vi "Autonomous No Shift 1 Tote 1 Container.vi"(11 "Cluster":T2={"Move Speed"=0.0, "Turning Speed"=0.53, "Arm speed"=0.0, "Desired Arm height (lift)"=17.0, "Initial Turn (Degrees)"=-18.0, "Desired Arm height (lowered)"=-12.0, "Drive Forward Time"=0.0, "Turn Degrees"=-130.0, "Position Speed"=0.3, "2nd Lift Height"=10.0}) -> ()   [LabVIEW 2014]
uses:
  Backup Auto States.ctl
  Robot Global Data.vi
  Desired Arm Position.vi
  <vilib>/Rock Robotics/WPI/RobotDrive/WPI_RobotDriveGetSetRefNum.vi
  <vilib>/Rock Robotics/WPI/RobotDrive/WPI_RobotDriveArcadeDrive_Standard(NoSaturation).vi
panel:
  in  "End Position?":bool
  out "Enum":T1=enum."Stop"
  in  "Range":dbl=2.0
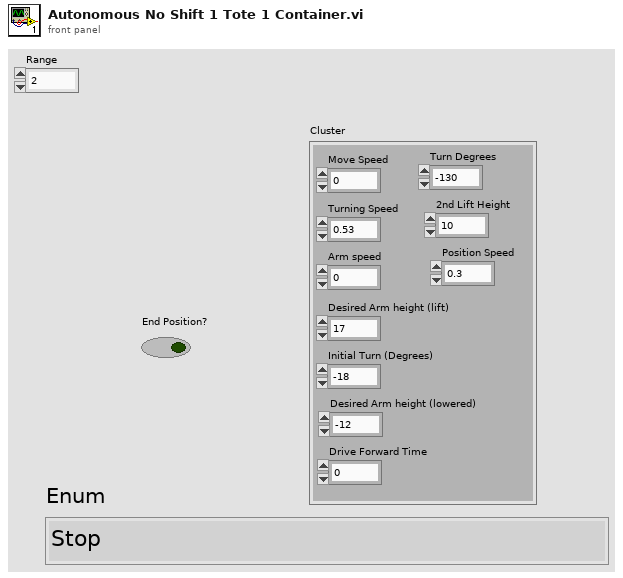
[diagram p1: front panel]
types:
  T1 = typedef "Backup Auto States.ctl" = enum16{"Start", "Grab container", "Lift arms", "Move to position", "Position robot", "Let go of container + Lower Arms", "Lift tote and container", "Turn towards S.P.", "Move forward", "Turn After hitting S.P.", "Move Until S.P. is gone", "Turn towards Auto Zone", "Drive to Auto Zone", "Stop"}
  T2 = cluster{"Move Speed":dbl, "Turning Speed":dbl, "Arm speed":dbl, "Desired Arm height (lift)":dbl, "Initial Turn (Degrees)":dbl, "Desired Arm height (lowered)":dbl, "Drive Forward Time":dbl, "Turn Degrees":dbl, "Position Speed":dbl, "2nd Lift Height":dbl}
  T3 = typedef "WPI_DigitalInputDevRef.ctl" = cluster{"DevStatus":errorcluster, "DIO Channel":T4, "Controller":T5}
  T4 = typedef "FPGA_DIOChannel.ctl" = enum8{"DIO 0", "DIO 1", "DIO 2", "DIO 3", "DIO 4", "DIO 5", "DIO 6", "DIO 7", "DIO 8", "DIO 9", "DIO MXP 0", "DIO MXP 1", "DIO MXP 2", "DIO MXP 3", "DIO MXP 4", "DIO MXP 5", "DIO MXP 6", "DIO MXP 7", "DIO MXP 8", "DIO MXP 9", "DIO MXP 10", "DIO MXP 11", "DIO MXP 12", "DIO MXP 13", "DIO MXP 14", "DIO MXP 15", "Invalid"}
  T5 = typedef "FPGA_TypedefDigitalModule.ctl" = enum16{"Controller 1"}
  T6 = typedef "WPI_RobotDriveDevRef.ctl" = cluster{"DevStatus":errorcluster, "Motors[]":T7[], "Square Inputs":bool, "Max Output":dbl}
  T7 = typedef "WPI_MotorControlDeviceRef.ctl" = cluster{"DeviceStatus":errorcluster, "Type":T8, "PWM":cluster{"Controller":T5, "PWM Channel":T9, "DeadBand":T10}, "CAN":cluster{"Device Number":u8, "Control Mode":T11, "Semaphore":T12, "Max Vout":dbl, "TalonSRX Control Mode":T13}, "Invert":bool, "TransformRef":T14, "InvTransformRef":T14}
  T8 = typedef "WPI_MotorControlType.ctl" = enum16{"PWM", "CAN", "CANTalonSRX"}
  T9 = typedef "FPGA_DIOPWMChannel.ctl" = enum8{"PWM 0", "PWM 1", "PWM 2", "PWM 3", "PWM 4", "PWM 5", "PWM 6", "PWM 7", "PWM 8", "PWM 9", "PWM MXP 0", "PWM MXP 1", "PWM MXP 2", "PWM MXP 3", "PWM MXP 4", "PWM MXP 5", "PWM MXP 6", "PWM MXP 7", "PWM MXP 8", "PWM MXP 9", "Invalid"}
  T10 = typedef "WPI_PWMDeadband.ctl" = cluster{"Name":string, "maxPositivePwm":i32, "minPositivePwm":i32, "centerPwm":i32, "maxNegativePwm":i32, "minNegativePwm":i32, "angularRange":u16}
  T11 = typedef "WPI_CANJaguar_ControlMode.ctl" = enum8{"Percent VBus", "Current", "Speed", "Position", "Voltage"}
  T12 = typedef "Semaphore RefNum" = refnum<k1>
  T13 = typedef "WPI_CANTalonSRX_APIControlMode.ctl" = enum8{"Percent VBus", "Speed", "Position", "Slave", "Unchanged / Invalid"}
  T14 = typedef "WPI_PWMTransform_ConPane.ctl" = refnum<vi>
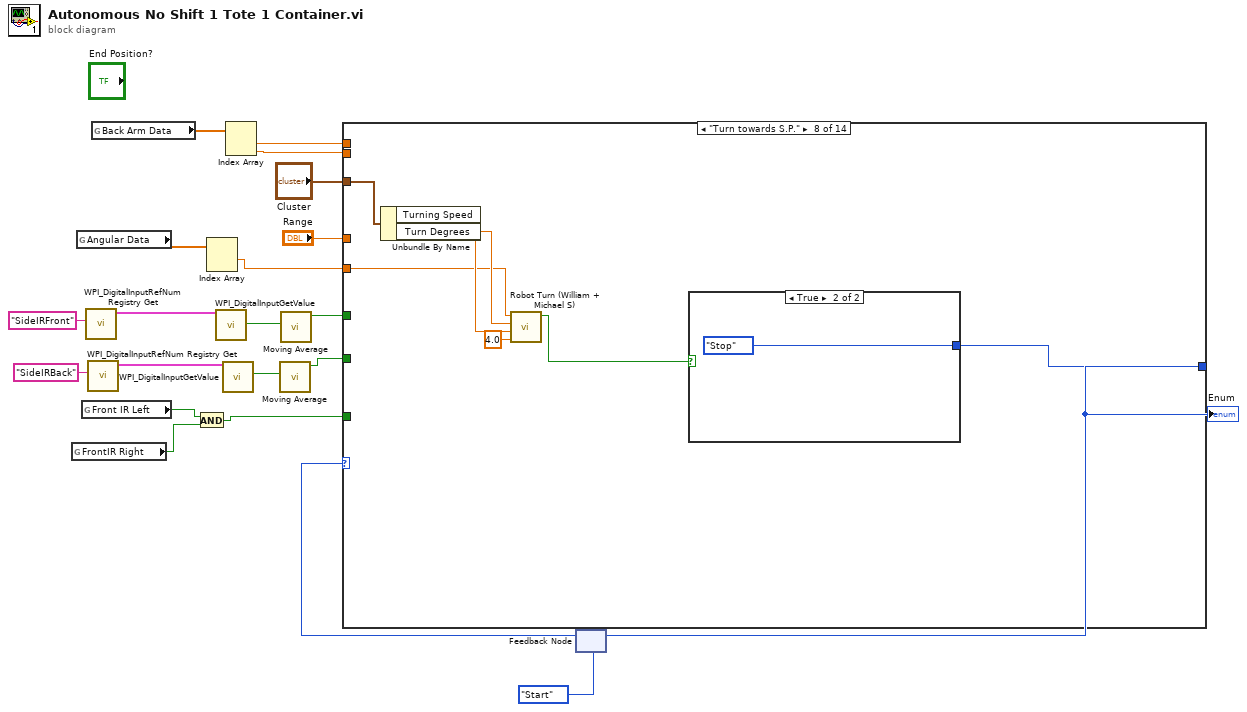
[diagram p0: block diagram]
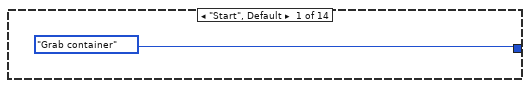
[diagram p2: hidden frame]
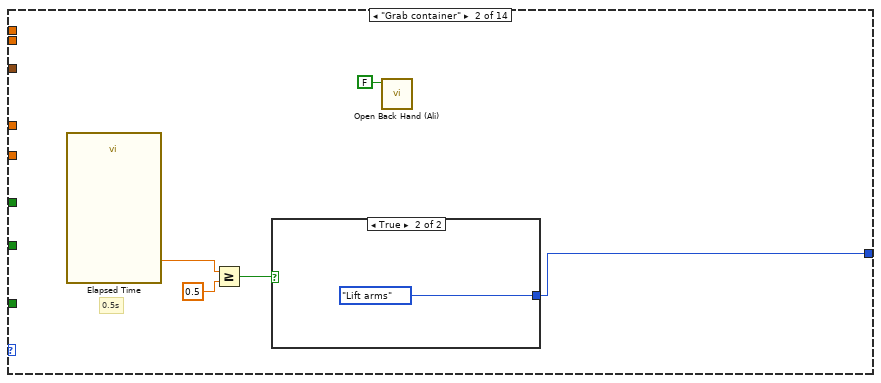
[diagram p3: hidden frame]
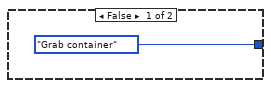
[diagram p4: hidden frame]
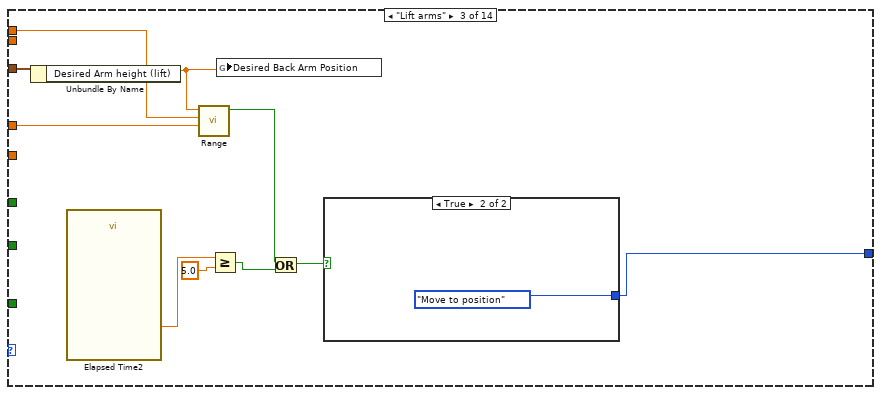
[diagram p5: hidden frame]
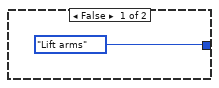
[diagram p6: hidden frame]
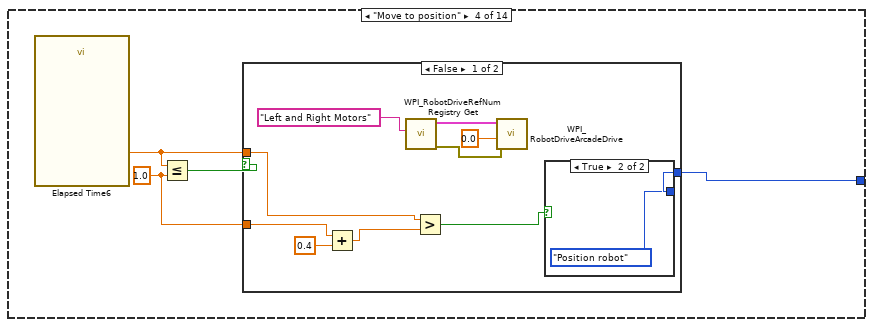
[diagram p7: hidden frame]
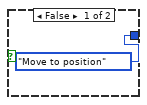
[diagram p8: hidden frame]
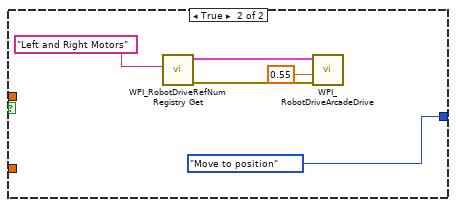
[diagram p9: hidden frame]
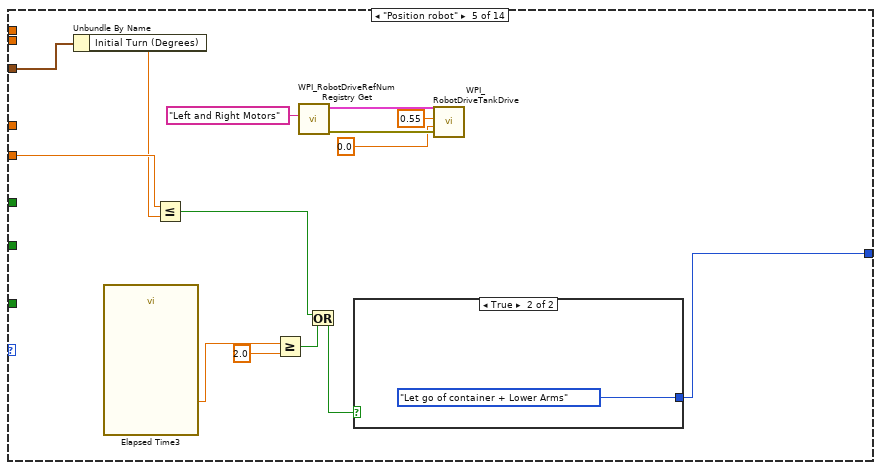
[diagram p10: hidden frame]
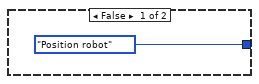
[diagram p11: hidden frame]
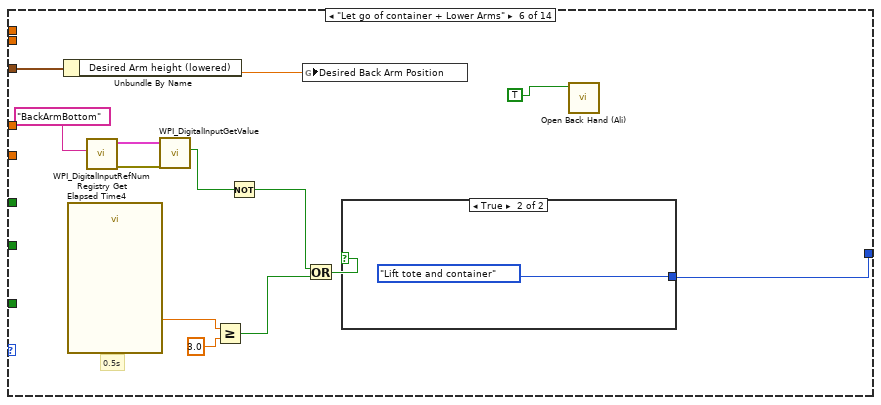
[diagram p12: hidden frame]
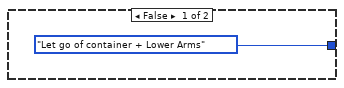
[diagram p13: hidden frame]
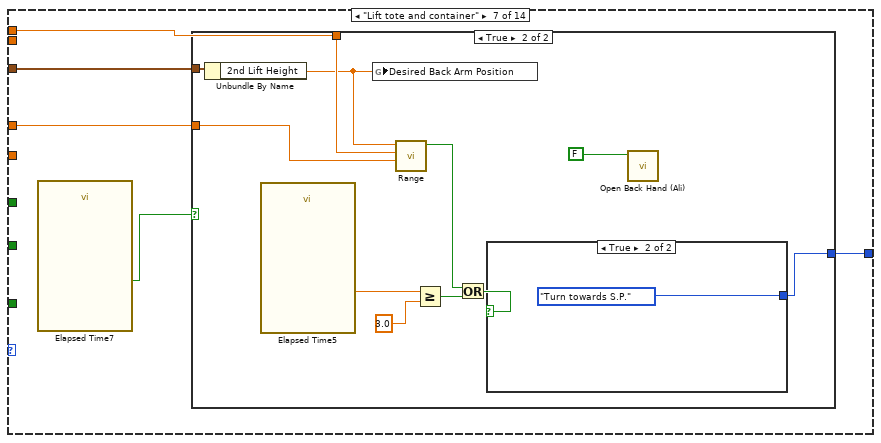
[diagram p14: hidden frame]
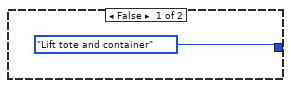
[diagram p15: hidden frame]
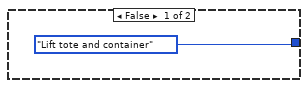
[diagram p16: hidden frame]
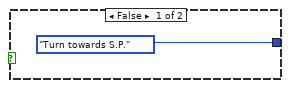
[diagram p17: hidden frame]
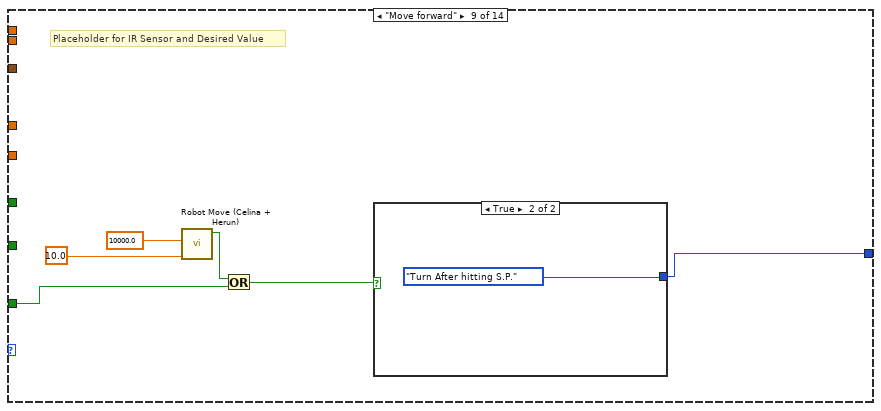
[diagram p18: hidden frame]
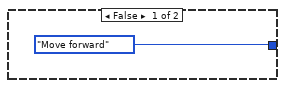
[diagram p19: hidden frame]
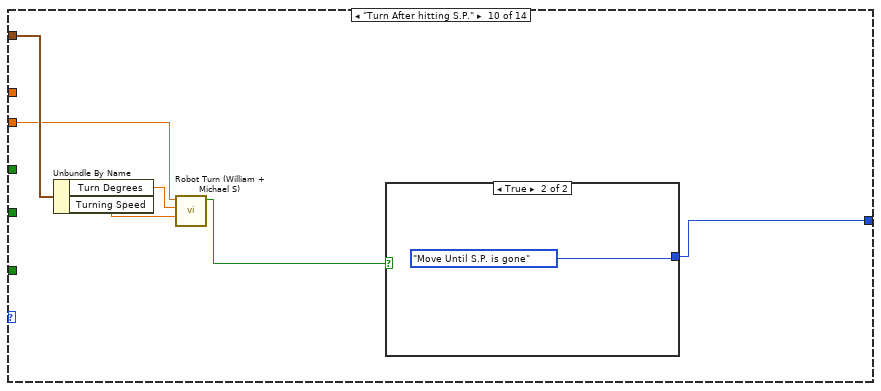
[diagram p20: hidden frame]
diagram:
  n1 = global read "Robot Global Data.vi" "FrontIR Right"() -> (w10:bool)
  n2 = global read "Robot Global Data.vi" "Angular Data"() -> (w14:dbl[])
  n3 = global read "Robot Global Data.vi" "Front IR Left"() -> (w11:bool)
  n4 = call <vilib>:"WPI_DigitalInputRefNum Registry Get.vi"("refnum name"="SideIRFront") -> ("DigitalInputDevRef"=w3:T3)  [unwired: 9 in, 1 out]
  n5 = call <vilib>:"WPI_DigitalInputRefNum Registry Get.vi"("refnum name"="SideIRBack") -> ("DigitalInputDevRef"=w4:T3)  [unwired: 9 in, 1 out]
  n6 = global read "Robot Global Data.vi" "Back Arm Data"() -> (w17:dbl[])
  n7 = And(x=w11, y=w10) -> (x .and. y?=w9:bool)
  n8 = Index Array(array=w14) -> (element #1=w13:dbl)  [unwired: 2 in, 1 out]
  n9 = call <vilib>:"WPI_DigitalInputGetValue.vi"("DigitalInputDevRef"=w3) -> ("Value"=w6:bool)  [unwired: 8 in, 2 out]
  n10 = call <vilib>:"WPI_DigitalInputGetValue.vi"("DigitalInputDevRef"=w4) -> ("Value"=w5:bool)  [unwired: 8 in, 2 out]
  n11 = Index Array(array=w17) -> (element #1=w16:dbl, element #2=w15:dbl)  [unwired: 2 in]
  n12 = call "Moving Average.vi"("Value"=w5) -> ("Moving Boolean Average"=w2:bool)  [unwired: 10 in]
  n13 = call "Moving Average.vi"("Value"=w6) -> ("Moving Boolean Average"=w1:bool)  [unwired: 10 in]
  n14 = feedback #1(Backup_Auto_States."Start" ("Enum")) -> (w19:T1)
  n15 = case shown="\"Turn towards S.P.\"" w19 {
    tunnel: "Cluster" -> [_ _ w31 _ w74 w85 w97 w119 _ w134 w147 w156 w162 _]
    tunnel: [Backup_Auto_States."Grab container" ("Enum") w23 w35 w44 w73 w86 w98 w115 w124 w135 w145 w151 w163 Backup_Auto_States."Stop" ("Enum")] -> w18
    tunnel: w9 -> [_ _ _ _ _ _ _ _ w123 _ _ _ _ _]
    tunnel: w16 -> [_ _ w34 _ _ _ w96 _ _ _ _ _ _ _]
    tunnel: w15 -> [_ _ _ _ _ _ _ _ _ _ _ _ _ _]
    tunnel: w13 -> [_ _ _ _ w69 _ _ w114 _ w130 _ w150 _ _]
    tunnel: "Range" -> [_ _ w32 _ _ _ w95 _ _ _ _ _ _ _]
    tunnel: w2 -> [_ _ _ _ _ _ _ _ _ _ w142 _ _ _]
    tunnel: w1 -> [_ _ _ _ _ _ _ _ _ _ w141 _ _ _]
    frame "Start", Default {
    }
    frame "Grab container" {
      # "0.5s"
      n16 = call "Elapsed Time"() -> ("Elapsed Time (s)"=w27:dbl)  [unwired: 12 in, 7 out]
      n17 = Greater Or Equal?(x=w27, y=0.5) -> (x >= y?=w25:bool)
      n18 = case shown="True" w25 {
        tunnel: [Backup_Auto_States."Grab container" ("Enum") Backup_Auto_States."Lift arms" ("Enum")] -> w23
        frame False {
        }
        frame True {
        }
      }
      n19 = call "Open Back Hand (Ali).vi"("Open?"=FALSE) -> ()  [unwired: 11 in]
    }
    frame "Lift arms" {
      n20 = Unbundle By Name(w31) -> ("Desired Arm height (lift)"=w30:dbl)
      n21 = call "Elapsed Time2"() -> ("Elapsed Time (s)"=w39:dbl)  [unwired: 12 in, 7 out]
      n22 = call "Range.vi"("Range"=w32, "Input"=w34, "In Range of"=w30) -> ("In Range?"=w33:bool)  [unwired: 8 in]
      n23 = Greater Or Equal?(x=w39, y=5.0) -> (x >= y?=w37:bool)
      n24 = global write "Desired Arm Position.vi" "Desired Back Arm Position"(w30) -> ()
      n25 = Or(x=w33, y=w37) -> (x .or. y?=w36:bool)
      n26 = case shown="True" w36 {
        tunnel: [Backup_Auto_States."Lift arms" ("Enum") Backup_Auto_States."Move to position" ("Enum")] -> w35
        frame False {
        }
        frame True {
        }
      }
    }
    frame "Move to position" {
      w42 = 1.0 ("y")
      n27 = call "Elapsed Time6"() -> ("Elapsed Time (s)"=w43:dbl)  [unwired: 12 in, 7 out]
      n28 = Less Or Equal?(x=w43, y=w42) -> (x <= y?=w45:bool)
      n29 = case shown="False" w45 {
        tunnel: [w51 Backup_Auto_States."Move to position" ("Enum")] -> w44
        tunnel: w43 -> [w50 _]
        tunnel: w42 -> [w48 _]
        frame False {
          n30 = Add(x=w48, y=0.4) -> (x+y=w46:dbl)
          n31 = call <vilib>:"WPI_RobotDriveRefNum Registry Get.vi"("refnum name"="Left and Right Motors") -> ("error out"=w54:errorcluster, "RobotDriveDevRef"=w52:T6)  [unwired: 9 in]
          n32 = Greater?(x=w50, y=w46) -> (0:w49:bool)
          n33 = call-poly <vilib>:"WPI_RobotDriveArcadeDrive.vi"("error in (no error)"=w54, "Y axis value"=0.0, "RobotDriveDevRef"=w52) -> ()  [unwired: 6 in, 3 out]
          n34 = case shown="True" w49 {
            tunnel: [Backup_Auto_States."Move to position" ("Enum") Backup_Auto_States."Position robot" ("Enum")] -> w51
            frame False {
            }
            frame True {
            }
          }
        }
        frame True {
          n35 = call <vilib>:"WPI_RobotDriveRefNum Registry Get.vi"("refnum name"="Left and Right Motors") -> ("error out"=w61:errorcluster, "RobotDriveDevRef"=w62:T6)  [unwired: 9 in]
          n36 = call-poly <vilib>:"WPI_RobotDriveArcadeDrive.vi"("error in (no error)"=w61, "Y axis value"=0.55, "RobotDriveDevRef"=w62) -> ()  [unwired: 6 in, 3 out]
        }
      }
    }
    frame "Position robot" {
      n37 = Unbundle By Name(w74) -> ("Initial Turn (Degrees)"=w68:dbl)
      n38 = call "Elapsed Time3"() -> ("Elapsed Time (s)"=w76:dbl)  [unwired: 12 in, 7 out]
      n39 = Less Or Equal?(x=w69, y=w68) -> (x <= y?=w66:bool)
      n40 = Greater Or Equal?(x=w76, y=2.0) -> (x >= y?=w67:bool)
      n41 = call <vilib>:"WPI_RobotDriveRefNum Registry Get.vi"("refnum name"="Left and Right Motors") -> ("error out"=w71:errorcluster, "RobotDriveDevRef"=w72:T6)  [unwired: 9 in]
      n42 = Or(x=w66, y=w67) -> (x .or. y?=w65:bool)
      n43 = case shown="True" w65 {
        tunnel: [Backup_Auto_States."Position robot" ("Enum") Backup_Auto_States."Let go of container + Lower Arms" ("Enum")] -> w73
        frame False {
        }
        frame True {
        }
      }
      n44 = call <vilib>:"WPI_RobotDriveTankDrive.vi"("error in (no error)"=w71, "Right axis value"=0.0 ("Left axis value"), "Left axis value"=0.55, "RobotDriveDevRef"=w72) -> ()  [unwired: 5 in, 3 out]
    }
    frame "Let go of container + Lower Arms" {
      # "0.5s"
      n45 = Unbundle By Name(w85) -> ("Desired Arm height (lowered)"=w84:dbl)
      n46 = call "Elapsed Time4"() -> ("Elapsed Time (s)"=w89:dbl)  [unwired: 12 in, 7 out]
      n47 = call <vilib>:"WPI_DigitalInputRefNum Registry Get.vi"("refnum name"="BackArmBottom") -> ("error out"=w82:errorcluster, "DigitalInputDevRef"=w83:T3)  [unwired: 9 in]
      n48 = call <vilib>:"WPI_DigitalInputGetValue.vi"("error in (no error)"=w82, "DigitalInputDevRef"=w83) -> ("Value"=w80:bool)  [unwired: 7 in, 2 out]
      n49 = Greater Or Equal?(x=w89, y=3.0) -> (x >= y?=w91:bool)
      n50 = Not(x=w80) -> (.not. x?=w79:bool)
      n51 = global write "Desired Arm Position.vi" "Desired Back Arm Position"(w84) -> ()
      n52 = Or(x=w79, y=w91) -> (x .or. y?=w87:bool)
      n53 = case shown="True" w87 {
        tunnel: [Backup_Auto_States."Let go of container + Lower Arms" ("Enum") Backup_Auto_States."Lift tote and container" ("Enum")] -> w86
        frame False {
        }
        frame True {
        }
      }
      n54 = call "Open Back Hand (Ali).vi"("Open?"=TRUE) -> ()  [unwired: 11 in]
    }
    frame "Lift tote and container" {
      n55 = call "Elapsed Time7"() -> ("Time has Elapsed"=w94:bool)  [unwired: 12 in, 7 out]
      n56 = case shown="True" w94 {
        tunnel: [Backup_Auto_States."Lift tote and container" ("Enum") w105] -> w98
        tunnel: w97 -> [_ w104]
        tunnel: w96 -> [_ w103]
        tunnel: w95 -> [_ w100]
        frame False {
        }
        frame True {
          n57 = Unbundle By Name(w104) -> ("2nd Lift Height"=w102:dbl)
          n58 = call "Elapsed Time5"() -> ("Elapsed Time (s)"=w109:dbl)  [unwired: 12 in, 7 out]
          n59 = global write "Desired Arm Position.vi" "Desired Back Arm Position"(w102) -> ()
          n60 = call "Range.vi"("Range"=w100, "Input"=w103, "In Range of"=w102) -> ("In Range?"=w101:bool)  [unwired: 8 in]
          n61 = Greater Or Equal?(x=w109, y=3.0) -> (x >= y?=w107:bool)
          n62 = Or(x=w101, y=w107) -> (x .or. y?=w106:bool)
          n63 = case shown="True" w106 {
            tunnel: [Backup_Auto_States."Lift tote and container" ("Enum") Backup_Auto_States."Turn towards S.P." ("Enum")] -> w105
            frame False {
            }
            frame True {
            }
          }
          n64 = call "Open Back Hand (Ali).vi"("Open?"=FALSE) -> ()  [unwired: 11 in]
        }
      }
    }
    frame "Turn towards S.P." {
      n65 = Unbundle By Name(w119) -> ("Turning Speed"=w118:dbl, "Turn Degrees"=w117:dbl)
      n66 = call "Robot Turn (William + Michael S).vi"("Desired Time"=4.0, "X axis value"=w118, "Desired Degree"=w117, "Gyro Degrees"=w114) -> ("Stop"=w116:bool)  [unwired: 7 in]
      n67 = case shown="True" w116 {
        tunnel: [Backup_Auto_States."Turn towards S.P." ("Enum") Backup_Auto_States."Stop" ("Enum")] -> w115
        frame False {
        }
        frame True {
        }
      }
    }
    frame "Move forward" {
      # "Placeholder for IR Sensor and Desired Value"
      n68 = call "Robot Move (Celina + Herun).vi"("Desired Time"=10.0, "Desired Distance (ft)"=10000.0) -> ("Stop State"=w122:bool)  [unwired: 9 in]
      n69 = Or(x=w122, y=w123) -> (x .or. y?=w127:bool)
      n70 = case shown="True" w127 {
        tunnel: [Backup_Auto_States."Move forward" ("Enum") Backup_Auto_States."Turn After hitting S.P." ("Enum")] -> w124
        frame False {
        }
        frame True {
        }
      }
    }
    frame "Turn After hitting S.P." {
      n71 = Unbundle By Name(w134) -> ("Turn Degrees"=w133:dbl, "Turning Speed"=w132:dbl)
      n72 = call "Robot Turn (William + Michael S).vi"("X axis value"=w132, "Desired Degree"=w133, "Gyro Degrees"=w130) -> ("Stop"=w131:bool)  [unwired: 8 in]
      n73 = case shown="True" w131 {
        tunnel: [Backup_Auto_States."Turn After hitting S.P." ("Enum") Backup_Auto_States."Move Until S.P. is gone" ("Enum")] -> w135
        frame False {
        }
        frame True {
        }
      }
    }
    frame "Move Until S.P. is gone" {
      n74 = And(x=w141, y=w142) -> (x .and. y?=w140:bool)
      n75 = Not(x=w140) -> (.not. x?=w139:bool)
      n76 = Unbundle By Name(w147) -> ("Move Speed"=w144:dbl)
      n77 = call "Robot Move (with Controllers).vi"("Time Target"=10.0 ("Time Target (s)"), "Speed"=w144) -> ("Stop?"=w138:bool)  [unwired: 9 in]
      n78 = Or(x=w138, y=w139) -> (x .or. y?=w146:bool)
      n79 = case shown="True" w146 {
        tunnel: [Backup_Auto_States."Move Until S.P. is gone" ("Enum") Backup_Auto_States."Turn towards Auto Zone" ("Enum")] -> w145
        frame False {
        }
        frame True {
        }
      }
    }
    frame "Turn towards Auto Zone" {
      n80 = Unbundle By Name(w156) -> ("Turning Speed"=w155:dbl, "Turn Degrees"=w153:dbl)
      n81 = Negate(x=w153) -> (-x=w154:dbl)
      n82 = call "Robot Turn (William + Michael S).vi"("X axis value"=w155, "Desired Degree"=w154, "Gyro Degrees"=w150) -> ("Stop"=w152:bool)  [unwired: 8 in]
      n83 = case shown="True" w152 {
        tunnel: [Backup_Auto_States."Turn towards Auto Zone" ("Enum") Backup_Auto_States."Drive to Auto Zone" ("Enum")] -> w151
        frame False {
        }
        frame True {
        }
      }
    }
    frame "Drive to Auto Zone" {
      n84 = Unbundle By Name(w162) -> ("Move Speed"=w161:dbl, "Drive Forward Time"=w160:dbl)
      n85 = call "Robot Move (with Controllers).vi"("Time Target"=w160, "Speed"=w161) -> ("Stop?"=w159:bool)  [unwired: 9 in]
      n86 = case shown="True" w159 {
        tunnel: [Backup_Auto_States."Drive to Auto Zone" ("Enum") Backup_Auto_States."Stop" ("Enum")] -> w163
        frame False {
        }
        frame True {
        }
      }
    }
    frame "Stop" {
    }
  }
  "Enum" <- w18
  n87 = feedback-in #1(w18) -> ()
